vi "Disconnect.vi"(7 "error in (no error)":errorcluster, 10 "Gantry in":refnum<class "A3200.lvclass">) -> (0 "error out":errorcluster)   [LabVIEW 2016, in "A3200.lvclass"]
uses:
  A3200.lvclass
  A3200.lvclass/A3200.ctl
  Drivers/Aerotech A3200/Aerotech VIs.lvlib
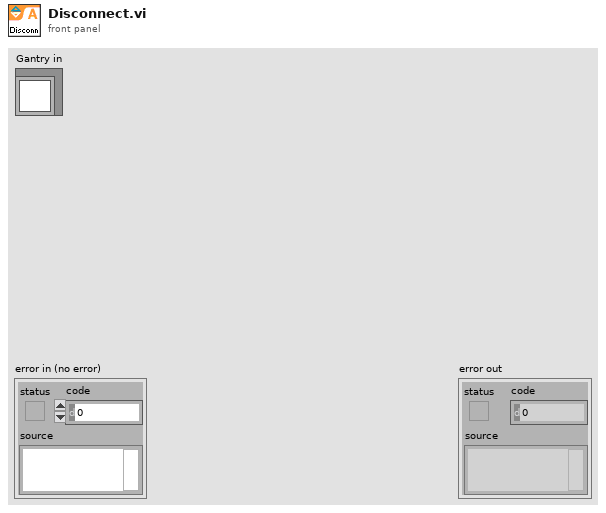
[diagram p1: front panel]
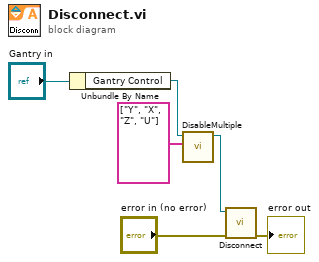
[diagram p0: block diagram]
diagram:
  n1 = Unbundle By Name("Gantry in") -> ("Gantry Control"=w3:refnum<k24>)
  n2 = call "DisableMultiple.vi"("axis names"=string[] ["Y", "X", "Z", "U"], "controller in"=w3) -> ("controller out"=w2:refnum<k24>)  [unwired: 8 in, 1 out]
  n3 = call "Disconnect.vi"("error in (no error)"="error in (no error)", "controller"=w2) -> ("error out"=→"error out":errorcluster)  [unwired: 9 in]
